vi "LED before trigger.vi"() -> ()   [LabVIEW 2016]
uses:
  <vilib>/MakerHub/LINX/Public/Peripherals/Digital/Digital Write 1 Chan.vi
  <vilib>/MakerHub/LINX/Public/Peripherals/Digital/Digital Write N Chans.vi
  <vilib>/MakerHub/LINX/Private/Local IO/LinxDigitalWrite.vi
  <vilib>/MakerHub/LINX/Public/Utilities/Check Channel.vi
  <vilib>/MakerHub/LINX/Public/Utilities/Open Serial.vi
  <vilib>/MakerHub/LINX/Private/Utilties/Generate Error.vi
  <vilib>/MakerHub/LINX/LMH-LINX.lvlib
panel:
  out "Time degree":dbl
  out "Time":dbl
  in  "Serial Port":refnum<visa-resource-name>="N/A"
  out "Boolean":bool
  in  "stop":bool
  in  "grados":i32=2 min=1 step=1
  in  "start":bool
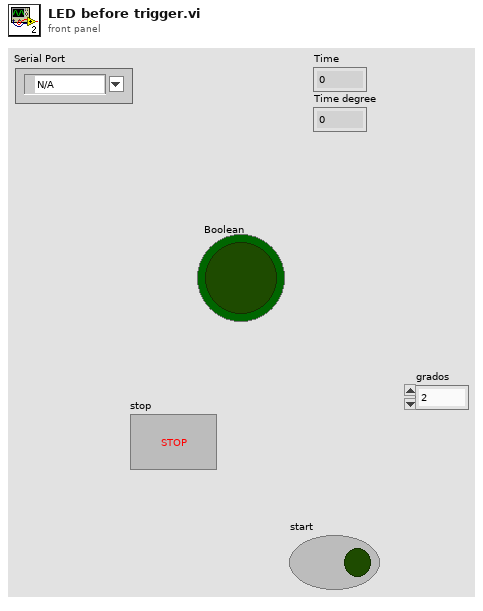
[diagram p1: front panel]
types:
  T1 = typedef "LMH-LINX.lvlib/LINX Ref.ctl" = cluster{"IO":T2, "Interface":T3, "LINX Device Config":T4}
  T2 = typedef "LMH-LINX.lvlib/Platform.ctl" = enum16{"Remote", "Local"}
  T3 = typedef "LMH-LINX.lvlib/Interface.ctl" = enum16{"Serial", "TCP"}
  T4 = typedef "LMH-LINX.lvlib/Device.lvlib/LINX Device Config.ctl" = cluster{"Interface":T3, "COM Port":refnum<visa-resource-name>, "TCP Configuration":T5, "Device Family":u8, "Device ID":u8, "Device Name":string, "TCP Ref":refnum<k5>, "Channels":T6}
  T5 = typedef "LMH-LINX.lvlib/Device.lvlib/TCP Config.ctl" = cluster{"IP Address":string, "Port":u16}
  T6 = typedef "LMH-LINX.lvlib/Channels.ctl" = cluster{"DI":u8[], "DO":u8[], "AI":u8[], "AO":u8[], "PWM":u8[], "QE":u8[], "UART":u8[], "I2C 2":u8[], "SPI":u8[], "CAN":u8[], "Servo":u8[], "AI Ref (V)":dbl, "AI Resolution (Bits)":u8, "AO Ref (V)":dbl, "AO Resolution (Bits)":u8}
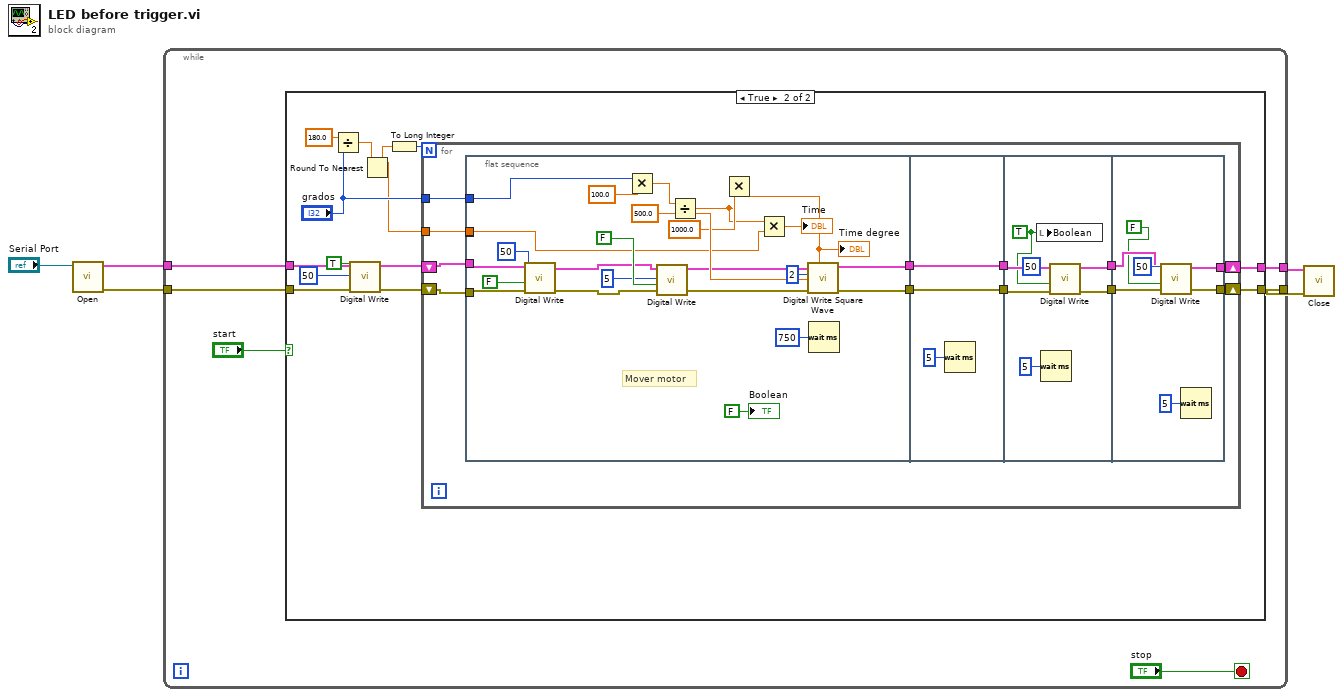
[diagram p0: block diagram]
diagram:
  n1 = call-poly <vilib>:"Open.vi"("Serial Port"="Serial Port") -> ("Error Out"=w4:errorcluster, "LINX Resource"=w5:T1)  [unwired: 8 in, 1 out]
  n2 = while {
    tunnel: w5 -> [w10]
    tunnel: w4 -> [w9]
    tunnel: [w8] -> w2
    tunnel: [w7] -> w3
    stop <- "stop" stop-if-true
    n3 = case shown="True" "start" {
      tunnel: w10 -> [w13 w16]
      tunnel: w9 -> [w12 w18]
      tunnel: [w12 w26] -> w8
      tunnel: [w13 w25] -> w7
      frame False {
      }
      frame True {
        n4 = Divide(x=180.0, y="grados") -> (x/y=w23:dbl)
        n5 = call-poly <vilib>:"Digital Write.vi"("Error In"=w18, "Output Value"=TRUE, "DO Channel"=u8 50, "LINX Resource"=w16) -> ("Error Out"=w19:errorcluster, "LINX Resource"=w15:T1)  [unwired: 6 in]
        n6 = Round To Nearest(number=w23) -> (nearest integer value=w20:dbl)
        n7 = To Long Integer(number=w20) -> (32bit integer=w22:i32)
        n8 = for {
          N: w22 -> [_]
          shift-right: [w28] -> w26
          shift-left: w19 -> [w38]
          shift-right: [w29] -> w25
          shift-left: w15 -> [w37]
          tunnel: "grados" -> [w30]
          tunnel: w20 -> [w27]
          n9 = flat-sequence {
            tunnel: w38 -> [w48]
            tunnel: w37 -> [w45]
            tunnel: [w52] -> w34
            tunnel: [w51] -> w31
            tunnel: w30 -> [w49]
            tunnel: [w40] -> _
            tunnel: w27 -> [w40]
            tunnel: [w65] -> w35
            tunnel: w34 -> [w65]
            tunnel: [w64] -> w32
            tunnel: w31 -> [w64]
            tunnel: [w70] -> w36
            tunnel: w35 -> [w71]
            tunnel: [w69] -> w33
            tunnel: w32 -> [w68]
            tunnel: w36 -> [w77]
            tunnel: w33 -> [w76]
            tunnel: [w75] -> w29
            tunnel: [w74] -> w28
            frame #0 {
              w58 = 500.0 ("y")
              # "Mover motor"
              n10 = call-poly <vilib>:"Digital Write.vi"("Error In"=w48, "Output Value"=FALSE, "DO Channel"=u8 50, "LINX Resource"=w45) -> ("Error Out"=w47:errorcluster, "LINX Resource"=w46:T1)  [unwired: 6 in]
              n11 = Multiply(x=w49, y=100.0) -> (x*y=w62:dbl)
              n12 = call-poly <vilib>:"Digital Write.vi"("Error In"=w47, "Output Value"=FALSE, "DO Channel"=u8 5, "LINX Resource"=w46) -> ("Error Out"=w55:errorcluster, "LINX Resource"=w56:T1)  [unwired: 6 in]
              n13 = Divide(x=w62, y=w58) -> (x/y=w41:dbl)
              n14 = Multiply(x=w41, y=1000.0) -> (x*y=w42:dbl)
              "Time degree" <- w42
              n15 = Multiply(x=w41, y=w40) -> (x*y=→"Time":dbl)
              n16 = call <vilib>:"Digital Write Square Wave.vi"("Duration (ms)"=w42, "Error In"=w55, "Frequency (Hz)"=w58, "Channel"=u8 2, "LINX Resource"=w56) -> ("Error Out"=w52:errorcluster, "LINX Resource"=w51:T1)  [unwired: 5 in]
              n17 = Wait (ms)(milliseconds to wait=u32 750) -> ()  [unwired: 1 out]
              "Boolean" <- FALSE ("Boolean")
            }
            frame #1 {
              n18 = Wait (ms)(milliseconds to wait=u32 5) -> ()  [unwired: 1 out]
            }
            frame #2 {
              w66 = TRUE ("Boolean")
              n19 = local write "Boolean"(w66) -> ()
              n20 = Wait (ms)(milliseconds to wait=u32 5) -> ()  [unwired: 1 out]
              n21 = call-poly <vilib>:"Digital Write.vi"("Error In"=w71, "Output Value"=w66, "DO Channel"=u8 50, "LINX Resource"=w68) -> ("Error Out"=w70:errorcluster, "LINX Resource"=w69:T1)  [unwired: 6 in]
            }
            frame #3 {
              n22 = call-poly <vilib>:"Digital Write.vi"("Error In"=w77, "Output Value"=FALSE ("Boolean"), "DO Channel"=u8 50, "LINX Resource"=w76) -> ("Error Out"=w74:errorcluster, "LINX Resource"=w75:T1)  [unwired: 6 in]
              n23 = Wait (ms)(milliseconds to wait=u32 5) -> ()  [unwired: 1 out]
            }
          }
        }
      }
    }
  }
  n24 = call <vilib>:"Close.vi"("Error In"=w2, "LINX Resource"=w3) -> ()  [unwired: 9 in, 1 out]
